vi "Demo Slider.vi"(8 "error in (no error)":errorcluster) -> (0 "error out":errorcluster)   [LabVIEW 2011]
uses:
  VIremote.llb/VIremoteEvent.ctl
  VIremote.llb/VIremoteFunction.ctl
panel:
  in  "Vert. Slider":dbl(slide) scale=0.0..10.0
  in  "Numeric":dbl format="%#.0f"
  in  "Slider UsePopup\n(or no mouse emulation)\nUpdateWhileChanging":i32(slide)=21 caption="Slider" scale=0.0..50.0
  in  "Slider":i32(slide)=21 scale=0.0..50.0
  in  "VIremoteEvent":T1=enum."Connection Closed"
  # "Sliders can be draged as normal when you use mouse emulation. Without emulation, or with UsePopup property, a native iOS slide will popup with a +- button and a textfield for keyboard entry. The slider will have the same range as the scale range and the +- button will increment/decrement with the data entry increment value."
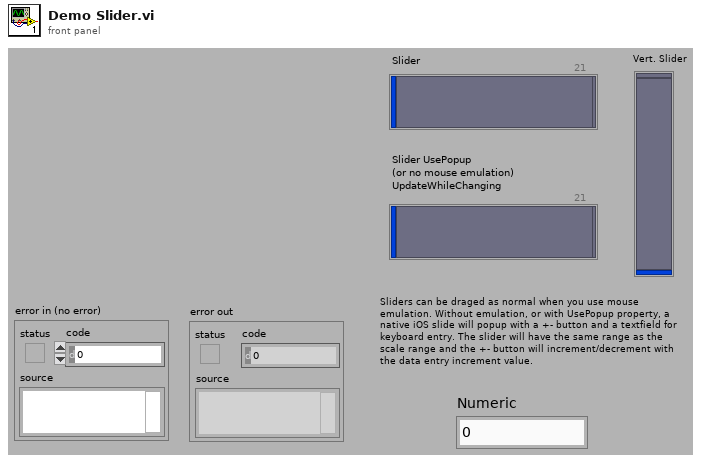
[diagram p1: front panel]
types:
  T1 = typedef "VIremoteEvent.ctl" = enum16{"No Event", "Connection Closed", "Navigate Back", "Enter Background", "Enter Foreground", "Portrait", "Portrait Upside Down", "Landscape Left", "Landscape Right"}
  T2 = typedef "VIremoteFunction.ctl" = enum16{"Do nothing", "Stop controller", "Close this connection", "Show info panel", "Set VI to control", "Set Accelerometer freq (Hz)", "Show Alert message", "Start Sound Input", "Stop Sound Input", "Set Volume (0-100)", "Set sound output Speaker", "Set sound output Receiver", "Play Sound", "Repeat Sound", "Stop Sound", "Pause Sound", "Resume Sound", "Set panel width of caller (320 or 480)", "Set Panel Size to Portrait", "Set Panel Size to Landscape", "Set Panel Size as Current Orientation", "Allow all UI Orientations", "Send user notification", "Disable Scrolling", "Normal Scrolling", "Page Scrolling", "Set Scroll Offset", "Page Indicator Position"}
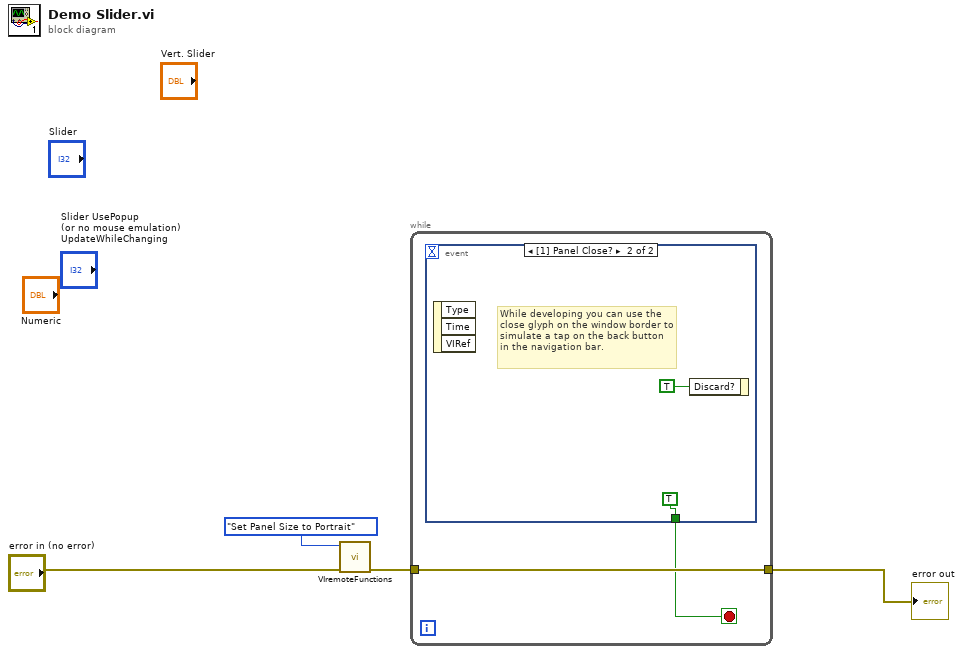
[diagram p0: block diagram]
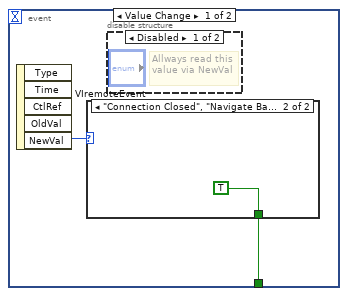
[diagram p2: hidden frame]
diagram:
  n1 = call "VIremoteFunctions.vi"("error in (no error)"="error in (no error)", "Function"=VIremoteFunction."Set Panel Size to Portrait") -> ("error out"=w3:errorcluster)  [unwired: 4 in, 5 out]
  n2 = while {
    tunnel: [w6] -> w1
    tunnel: w3 -> [w6]
    stop <- w5 stop-if-true
    n3 = event shown="[1] Panel Close?" {
      selector: _ -> [_ _]
      dyn-events: _ -> [_ _]
      timeout: _ -> [_ _]
      tunnel: [w7 TRUE] -> w5
      event Value Change {
        n4 = event-data() -> ("NewVal"=w8:T1)  [unwired: 5 out]
        n5 = case shown="\"Connection Closed\", \"Navigate Back\"" w8 {
          tunnel: [_ TRUE] -> w7
          frame "No Event", Default {
          }
          frame "Connection Closed", "Navigate Back" {
          }
        }
        n6 = disable-structure shown="Disabled" {
          frame Disabled {
            # "Allways read this value via NewVal"
          }
          frame Enabled {
          }
        }
      }
      event Panel Close? {
        # "While developing you can use the close glyph on the window border to simulate a tap on the back button in the navigation bar."
        n7 = event-data() -> ()  [unwired: 4 out]
        n8 = event-data("Discard?"=TRUE) -> ()  [unwired: 1 in, 1 out]
      }
    }
  }
  "error out" <- w1
